vi "To Serial Form.vi"(6 "Serial Version":T1, 10 "Serializer in":refnum<class "Serializer.lvclass">, 11 "CRDS in":refnum<class "CRDS.lvclass">) -> (0 "error out":errorcluster, 2 "Serializer out":refnum<class "Serializer.lvclass">, 3 "CRDS out":refnum<class "CRDS.lvclass">)   [LabVIEW 2012]
uses:
  <userlib>/Serialization/Serializable/Serializable.lvclass
  <userlib>/Serialization/Serializable/Insert Serializable.vi
  <userlib>/Serialization/Serializer/Serializer.lvclass
  <userlib>/Serialization/Serialization Common/Serial Version.ctl
  <userlib>/Serialization/Serialization Common/Serialization Common.lvlib
  CRDS.lvclass
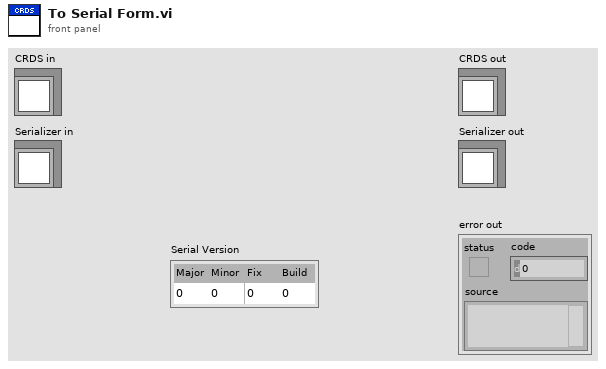
[diagram p1: front panel]
types:
  T1 = typedef "Serialization Common.lvlib/Serial Version.ctl" = cluster{"Major":u16, "Minor":u16, "Fix":u16, "Build":u16}
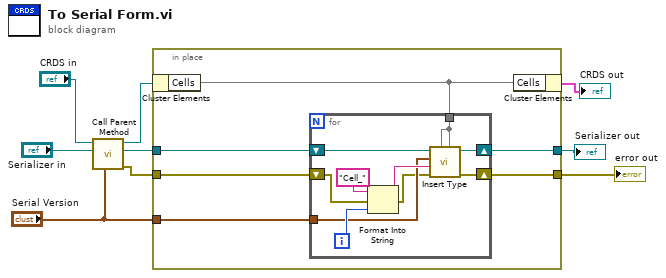
[diagram p0: block diagram]
diagram:
  n1 = call-parent "Call Parent Method"("Serial Version"="Serial Version", "Serializer in"="Serializer in", "Instrument in"="CRDS in") -> ("error out"=w4:errorcluster, "Serializer out"=w6:refnum<class "Serializer.lvclass">, "Instrument out"=w7:refnum<class "CRDS.lvclass">)  [unwired: 6 in]
  n2 = in-place {
    in-place-border: w6 -> [w14]
    in-place-border: "Serial Version" -> [w12]
    in-place-border: w4 -> [w13]
    in-place-border: [w11] -> w3
    in-place-border: [w10] -> w1
    n3 = in-place-cluster #1(w7) -> ("Cells"=w15)
    n4 = for {
      tunnel: w15 -> [w20]
      tunnel: w12 -> [w21]
      shift-right: [w18] -> w10
      shift-left: w13 -> [w17]
      shift-right: [w19] -> w11
      shift-left: w14 -> [w25]
      i -> [w24]
      n5 = Format Into String(initial string="Cell_", error in=w17, w24) -> (resulting string=w22:string, error out=w16:errorcluster)  [unwired: 1 in]
      n6 = call-poly <userlib>:"Insert Type.vi"("Serializable"=w20, "Default Value"=w20, "error in (no error)"=w16, "Name"=w22, "Serial Version"=w21, "Serializer in"=w25) -> ("error out"=w18:errorcluster, "Serializer out"=w19:refnum<class "Serializer.lvclass">)  [unwired: 4 in]
    }
    n7 = in-place-cluster #1("Cells"=w15) -> (→"CRDS out":cluster{})
  }
  "error out" <- w1
  "Serializer out" <- w3
